vi "test z counter.vi"() -> ()   [LabVIEW 2010]
uses:
  scan_specification_tagResonant.ctl
  counter_cluster_tagResonant.ctl
panel:
  out "acquire":bool
  in  "num reps":i32=10000
  out "trigger diagnostics":T1
  out "counter cluster out":T2
  in  "scan specification":T3={"z resolution (pixels)"=30, "iterations per pixel"=5, "iterations per z-scan (=zres*iterperpixel)"=150, "x resolution (pixels)"=80, "y resolution (pixels)"=80, "number of z-lines per volume"=5164, "number of repetitions (volumes)"=0, "Pockels cell voltage (bits)"=0, "Vx center (bits)"=0, "Vy center (bits)"=0, "Vx amplitude (bits)"=0, "Vy amplitude (bits)"=0, "lines to delay between scan start and output"=0, "LSB has acquire control"=FALSE}
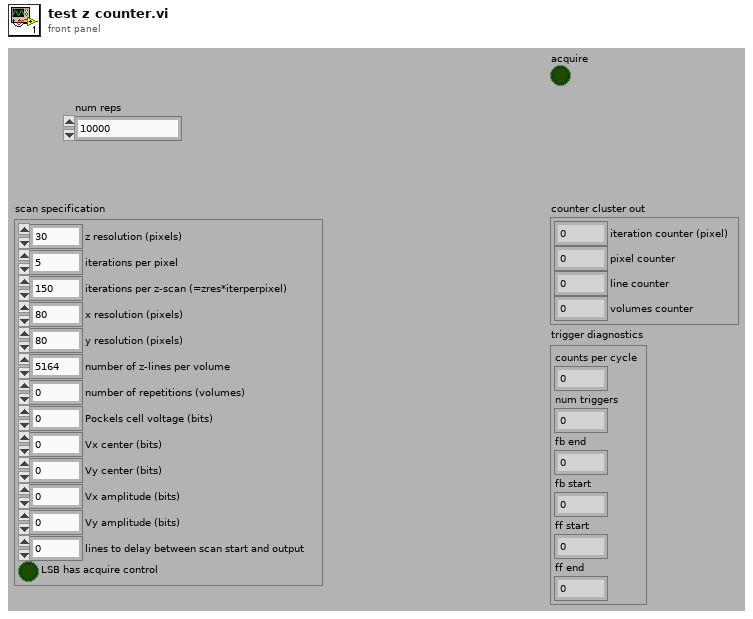
[diagram p1: front panel]
types:
  T1 = cluster{"counts per cycle":u16, "num triggers":u32, "fb end":u16, "fb start":u16, "ff start":u16, "ff end":u16}
  T2 = typedef "counter_cluster_tagResonant.ctl" = cluster{"iteration counter (pixel)":u16, "pixel counter":u16, "line counter":i16, "volumes counter":u16}
  T3 = typedef "scan_specification_tagResonant.ctl" = cluster{"z resolution (pixels)":u16, "iterations per pixel":u16, "iterations per z-scan (=zres*iterperpixel)":u16, "x resolution (pixels)":u16, "y resolution (pixels)":u16, "number of z-lines per volume":u16, "number of repetitions (volumes)":i32, "Pockels cell voltage (bits)":i16, "Vx center (bits)":i16, "Vy center (bits)":i16, "Vx amplitude (bits)":i16, "Vy amplitude (bits)":i16, "lines to delay between scan start and output":u16, "LSB has acquire control":bool}
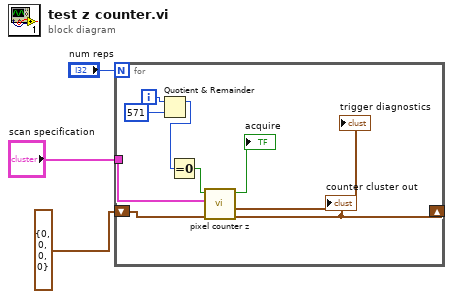
[diagram p0: block diagram]
diagram:
  n1 = for {
    N: "num reps" -> [_]
    tunnel: "scan specification" -> [w12]
    shift-right: [w11] -> _
    shift-left: T2 {"iteration counter (pixel)"=0, "pixel counter"=0, "line counter"=0, "volumes counter"=0} ("counter cluster out") -> [w9]
    i -> [w8]
    n2 = Quotient & Remainder(x=w8, y=571) -> (x-y*floor(x/y)=w6:i32)  [unwired: 1 out]
    n3 = Equal To 0?(x=w6) -> (x = 0?=w5:bool)
    n4 = call "pixel counter z.vi"("counter cluster in"=w9, "scan specification"=w12, "tag lens trigger"=w5) -> ("counter cluster out"=w11:T2, "trigger diagnostics"=→"trigger diagnostics":T1, "acquire"=→"acquire":bool)  [unwired: 4 in, 2 out]
    "counter cluster out" <- w11
  }
